vi "Settings.vi"(8 "error in (no error)":errorcluster, 11 "C4 Dispense in":refnum<class "Iterative Dispense.lvclass">) -> (0 "error out":errorcluster, 3 "C4 Dispense out":refnum<class "Iterative Dispense.lvclass">)   [LabVIEW 2020, in "Iterative Dispense.lvclass"]
uses:
  Iterative Dispense.lvclass
  C:/Users/hep/Documents/CMU gantry/Classes/Routine/Dispense/Dispense.lvclass
  Glue Step Enum.ctl
  Iterative Dispense.lvclass/Iterative Dispense.ctl
  Dispense.lvclass/Dispense.ctl
  Write Tip Height.vi
  Dispense.lvclass
panel:
  in  "Glue Step Enum":T1
  in  "Pattern":u16(ring) items=["Dodecagon", "Hexagon"]
  in  "Speed":dbl=30.0
  in  "Number of Lines":i32
  in  "Distance From Edges":dbl
  in  "PSI Low (*10)":i32 format="%1.0f"
  in  "PSI High (*10)":i32
  in  "Tip Height":dbl
  in  "Submit":bool=TRUE
  # "C4 Dispense"
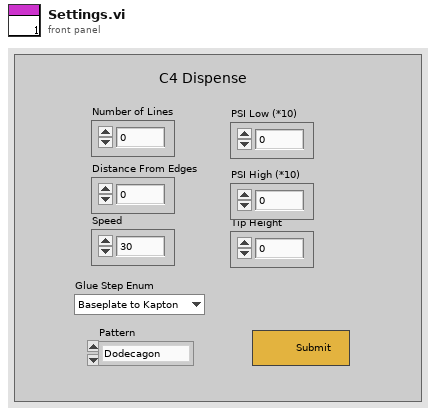
[diagram p1: front panel]
types:
  T1 = typedef "Iterative Dispense.lvclass/Glue Step Enum.ctl" = enum16{"Baseplate to Kapton", "Kapton to Sensor"}
  T2 = typedef "File Paths.ctl" = cluster{"Glue Pattern Folder":path, "Carrier Tray Folder":path, "Pick Up Tool Fixture Folder":path, "Components Folder":path, "Bellows Tool Offset.txt":path, "Pick Up Tool Offset.txt":path, "Dispense Tip Offset.txt":path, "Log Files":path}
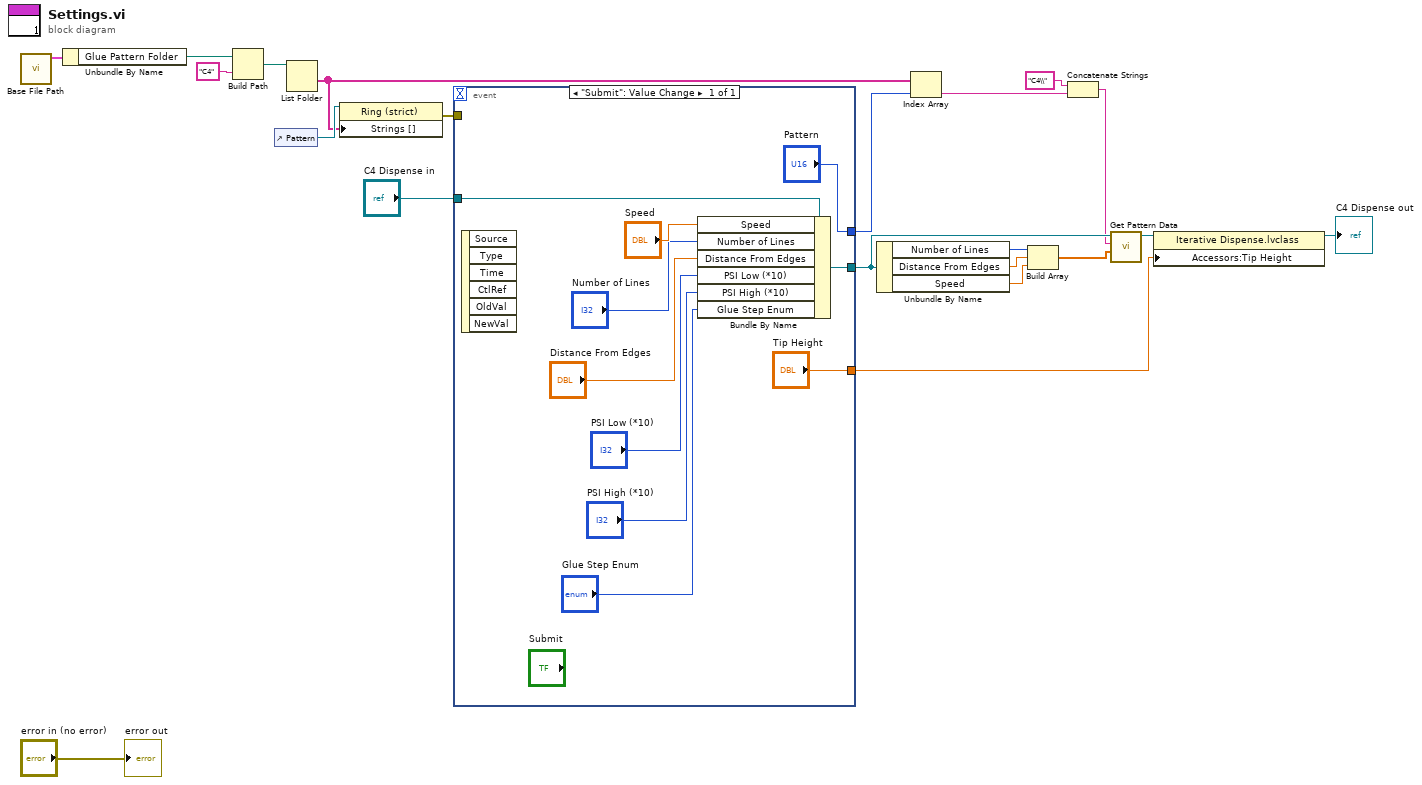
[diagram p0: block diagram]
diagram:
  n1 = call "Base File Path.vi"() -> ("Paths Out"=w17:T2)  [unwired: 11 in]
  n2 = Unbundle By Name(w17) -> ("Glue Pattern Folder"=w18:path)
  n3 = Build Path(base path=w18, name or relative path="C4") -> (appended path=w19:path)
  n4 = control-ref of="Pattern"() -> (w16:refnum<vi>)
  n5 = List Folder(path=w19) -> (folder names=w15:string[])  [unwired: 3 in, 3 out]
  n6 = property class="Ring (strict)"(reference=w16, "Strings []"=w15) -> (error out=w13:errorcluster)  [unwired: 1 in, 1 out]
  n7 = event shown="[0] \"Submit\": Value Change" {
    selector: _ -> [_]
    dyn-events: _ -> [_]
    timeout: _ -> [_]
    tunnel: "C4 Dispense in" -> [w31]
    tunnel: [w25] -> w8
    tunnel: ["Pattern"] -> w14
    tunnel: ["Tip Height"] -> w11
    tunnel: w13 -> [_]
    event "Submit": Value Change {
      n8 = event-data() -> ()  [unwired: 1 in, 6 out]
      n9 = Bundle By Name(cluster=w31, "Speed"="Speed", "Number of Lines"="Number of Lines", "Distance From Edges"="Distance From Edges", "PSI Low (*10)"="PSI Low (*10)", "PSI High (*10)"="PSI High (*10)", "Glue Step Enum"="Glue Step Enum") -> (w25:refnum<class "Iterative Dispense.lvclass">)
    }
  }
  n10 = Unbundle By Name(w8) -> ("Number of Lines"=w7:i32, "Distance From Edges"=w6:dbl, "Speed"=w5:dbl)
  n11 = Index Array(array=w15, index=w14) -> (element=w2:string)
  n12 = Build Array(w7, w6, w5) -> (w4:dbl[])
  n13 = Concatenate Strings("C4\\" ("string"), w2) -> (w1:string)
  n14 = call "Get Pattern Data.vi"("File Name"=w4, "Folder Name"=w1, "Dispense.lvclass"=w8) -> ("Dispense Out"=w10:refnum<class "Iterative Dispense.lvclass">)  [unwired: 8 in]
  n15 = property class="Iterative Dispense.lvclass"(reference=w10, "Accessors:Tip Height"=w11) -> (reference out=→"C4 Dispense out":refnum<class "Iterative Dispense.lvclass">)  [unwired: 1 in, 1 out]
  "error out" <- "error in (no error)"
